vi "SubTest Monitor - GTCP331-200ER.vi"(8 "error in (no error)":errorcluster, 11 "RT - Analysis Data in in":T1={"Accel Sensistivity"=[0.0, 0.0, 0.0], "Cutoff Frequncies"=[{"LP Passband"=0.0, "HP Stopband"=0.0, "LP Stopband"=0.0, "HP Passband"=0.0}, {"LP Passband"=0.0, "HP Stopband"=0.0, "LP Stopband"=0.0, "HP Passband"=0.0}, {"LP Passband"=0.0, "HP Stopband"=0.0, "LP Stopband"=0.0, "HP Passband"=0.0}], "APU Setup File"={"Sensor Info"=[], "Calibration Info"=[], "CMM Table 106"=[], "CMM Table 106B "=[], "Accel Config"=[], "Report Sheet 1"=[], "Report Sheet 2"=[], "Report Sheet 3"=[]}, "RepairLevel"=""} {"Cutoff Frequncies"."HP Passband" min=1.0 step=1.0 format="%#.4f"; "Cutoff Frequncies"."LP Stopband" min=1.0 step=1.0 format="%#.4f"; "Cutoff Frequncies"."HP Stopband" min=1.0 step=1.0 format="%#.4f"; "Cutoff Frequncies"."LP Passband" min=1.0 step=1.0 format="%#.4f"}) -> (0 "error out":errorcluster, 3 "RT - Analysis Data out":T1 {"Cutoff Frequncies"."HP Passband" min=1.0 step=1.0 format="%#.4f"; "Cutoff Frequncies"."LP Stopband" min=1.0 step=1.0 format="%#.4f"; "Cutoff Frequncies"."HP Stopband" min=1.0 step=1.0 format="%#.4f"; "Cutoff Frequncies"."LP Passband" min=1.0 step=1.0 format="%#.4f"})   [LabVIEW 2018, in "RT - Analysis.lvlib"]
doc: "Monitors the data for the input SubTest for the named APU."
uses:
  RT - Analysis.lvlib
  Private Controls/RT-Analysis Data.ctl
  Modules/Testing UI 3/Private Controls/Cutoff Frequency.ctl
  Modules/Testing UI 3/Testing UI 3.lvlib
  Top Level/Shared Controls/APU Setup File.ctl
panel:
  # "Highpass Cutoff Frequency"
  # "Lowpass Cutoff Frequency"
  # "Highpass Cutoff Frequency"
  # "Lowpass Cutoff Frequency"
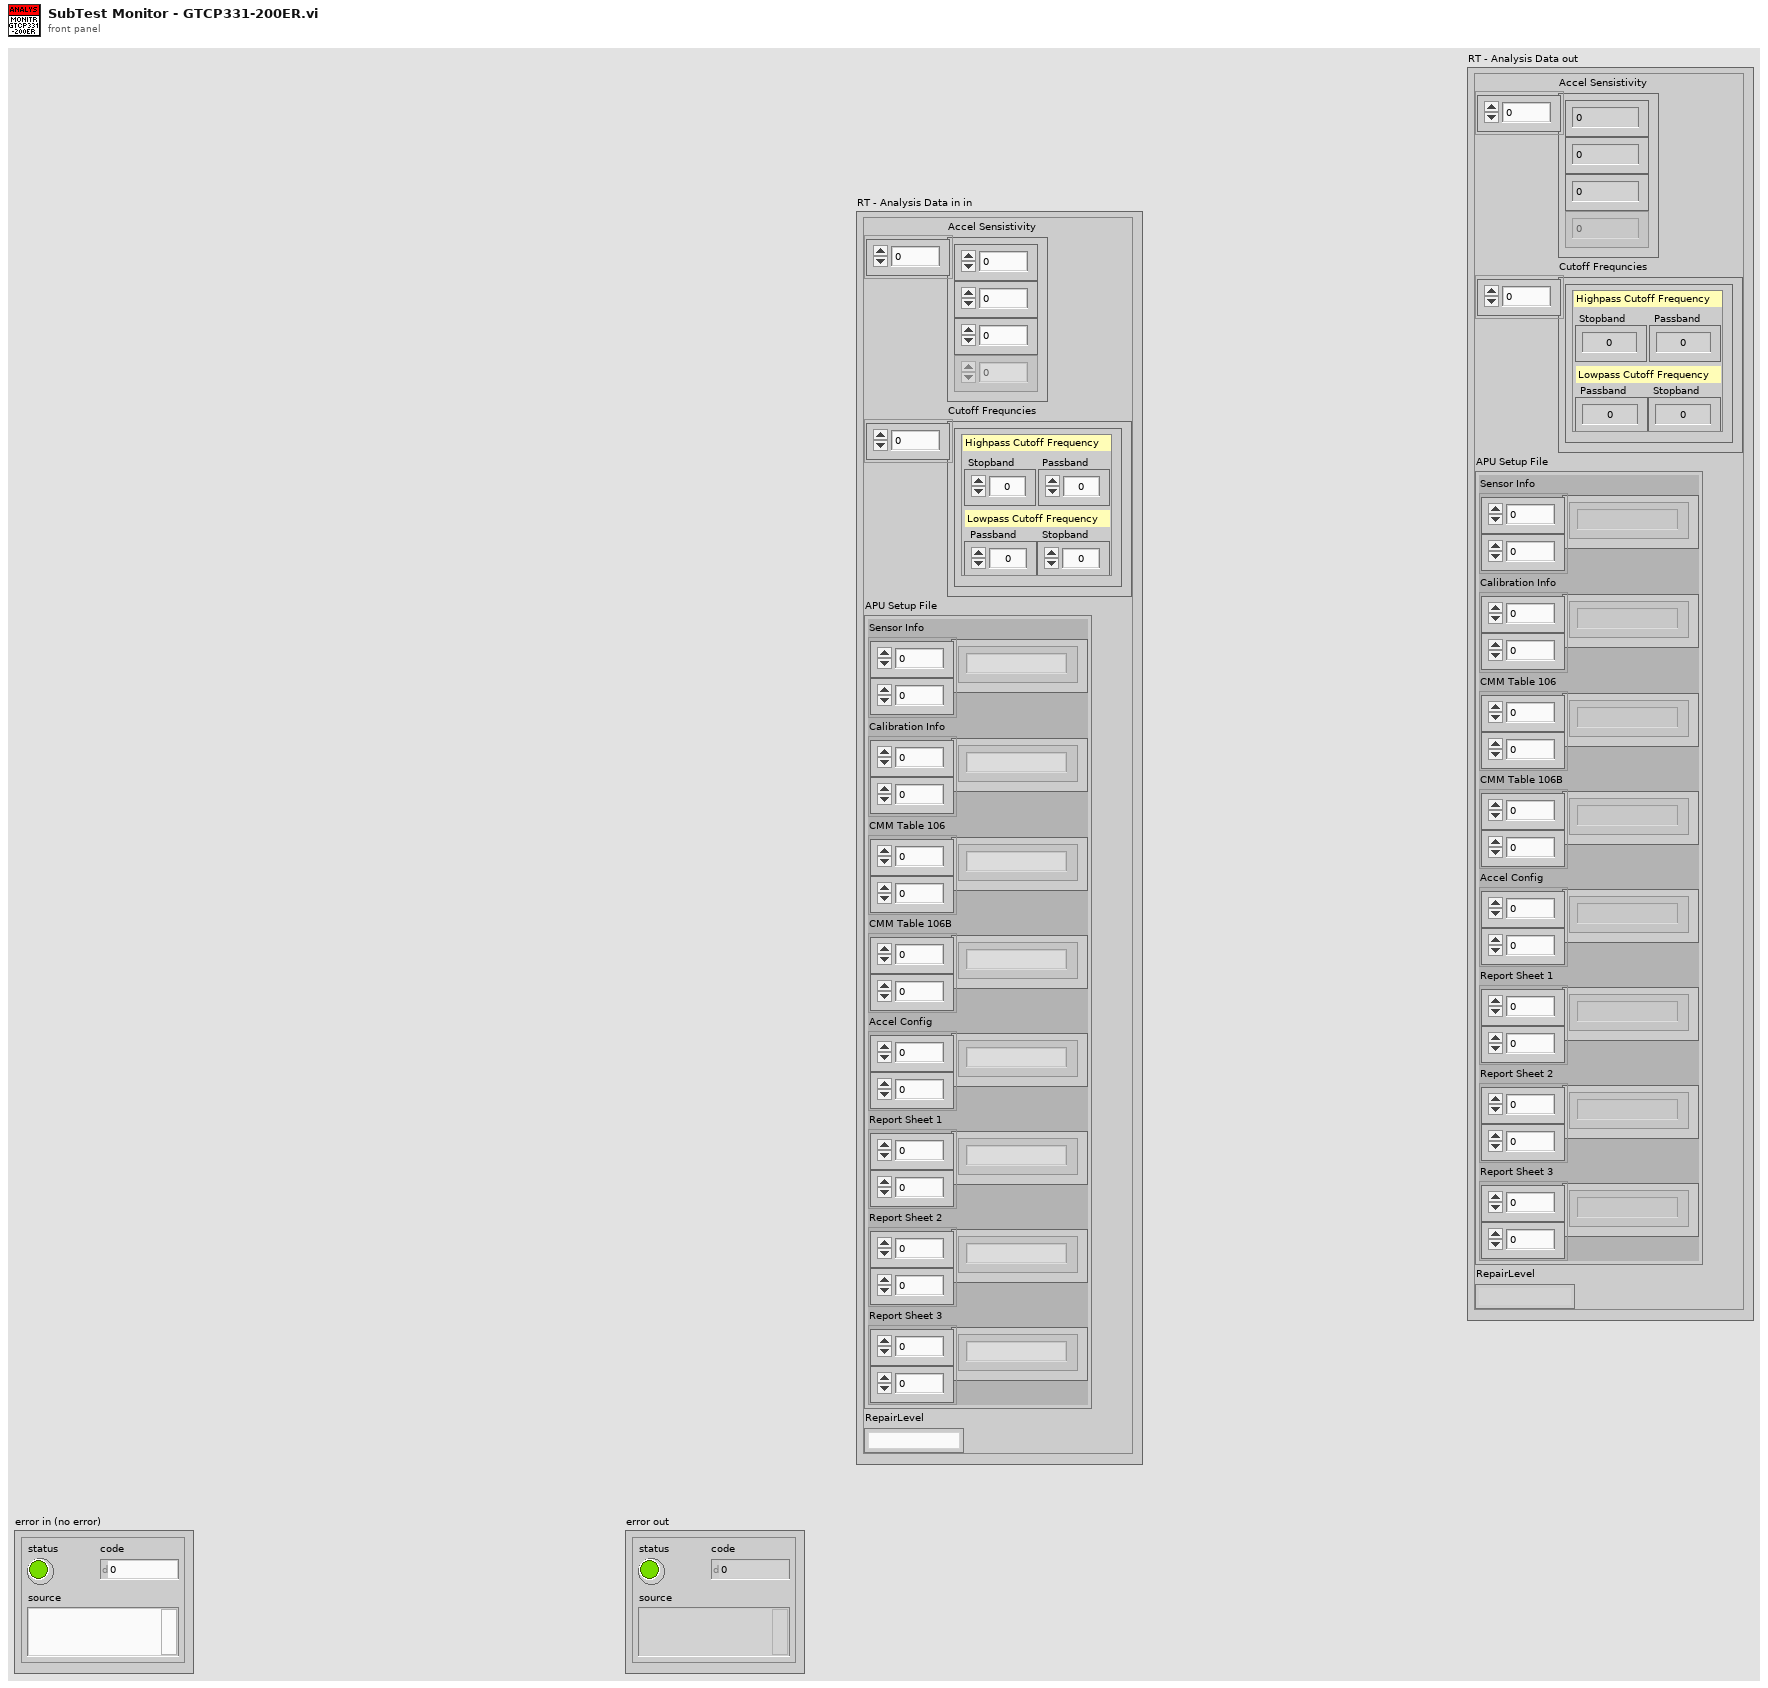
[diagram p1: front panel]
types:
  T1 = typedef "RT - Analysis.lvlib/RT-Analysis Data.ctl" = cluster{"Accel Sensistivity":dbl[], "Cutoff Frequncies":T2[], "APU Setup File":T3, "RepairLevel":string}
  T2 = typedef "Testing UI 3.lvlib/Cutoff Frequency.ctl" = cluster{"LP Passband":dbl, "HP Stopband":dbl, "LP Stopband":dbl, "HP Passband":dbl}
  T3 = typedef "APU Setup File.ctl" = cluster{"Sensor Info":string[][], "Calibration Info":string[][], "CMM Table 106":string[][], "CMM Table 106B ":string[][], "Accel Config":string[][], "Report Sheet 1":string[][], "Report Sheet 2":string[][], "Report Sheet 3":string[][]}
  T4 = typedef "Analyzed Data Sets.ctl" = T5[]
  T5 = typedef "All Data Cluster.ctl" = cluster{"Acq Data":T6, "Calculated Data":T7, "Indicator Data":cluster{"00-02-9234 Peak Vel (in/sec)":dbl[]}, "Calibrated Data":cluster{"00-00-9220 Calib":dbl[], "00-01-9220 Calib":dbl[], "02-03-9227 Calib":dbl[], "00-02-9234 Calib":dbl[], "02-05-9205 Calib":dbl[]}}
  T6 = typedef "Acq Data.ctl" = cluster{"00-00-9220":dbl[], "00-01-9220":dbl[], "01-00-9213":dbl[], "01-01-9213":dbl[], "01-02-9213":dbl[], "02-02-9219":dbl[], "02-03-9227":dbl[], "00-02-9234":dbl[], "00-03-9402":dbl[], "02-05-9205":dbl[], "02-04-9871":dbl[], "Timestamp":timestamp}
  T7 = typedef "Calculated Data.ctl" = cluster{"C.00":dbl, "C.01":dbl, "C.02":dbl, "C.03":dbl, "C.04":dbl, "C.05":dbl, "C.06":dbl, "C.07":dbl, "C.08":dbl, "C.09":dbl, "C.10":dbl, "C.11":dbl, "C.12":dbl, "C.13":dbl, "C.14":dbl, "C.15":dbl, "C.16":dbl, "C.17":dbl, "C.18":dbl, "C.19":dbl, "C.20":dbl, "C.21":dbl, "C.22":dbl, "C.23":dbl, "C.24":dbl, "C.25":dbl, "C.26":dbl, "C.27":dbl, "C.28":dbl, "C.29":dbl, "C.30":dbl, "C.31":dbl, "C.32":dbl, "C.33":dbl, "C.34":dbl, "C.35":dbl, "C.36":dbl, "C.37":dbl, "C.38":dbl, "C.39":dbl, "C.40":dbl, "C.41":dbl, "C.42":dbl, "C.43":dbl, "C.44":dbl, "C.45":dbl, "C.46":dbl, "C.47":dbl, "C.48":dbl, "C.49":dbl, "C.50":dbl, "C.51":dbl, "C.52":dbl, "C.53":dbl, "C.54":dbl, "C.56":dbl}
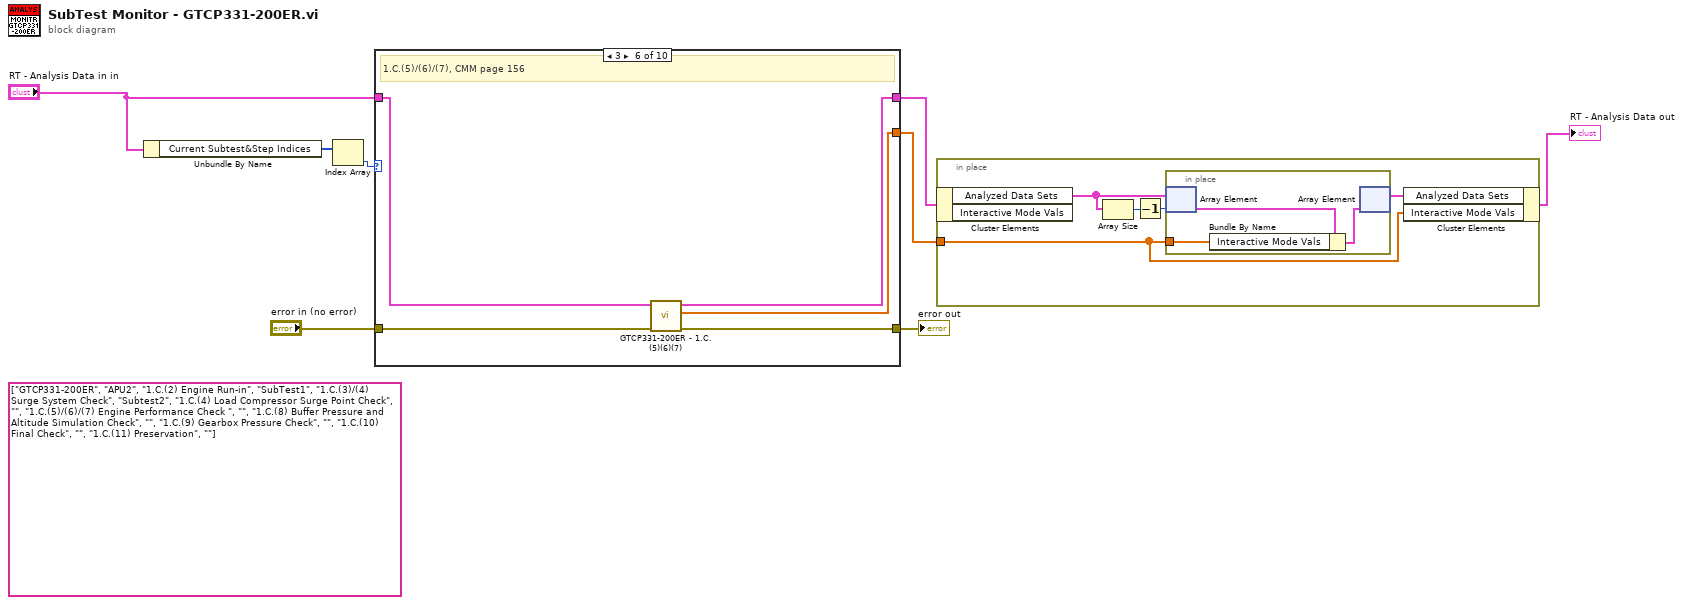
[diagram p0: block diagram]
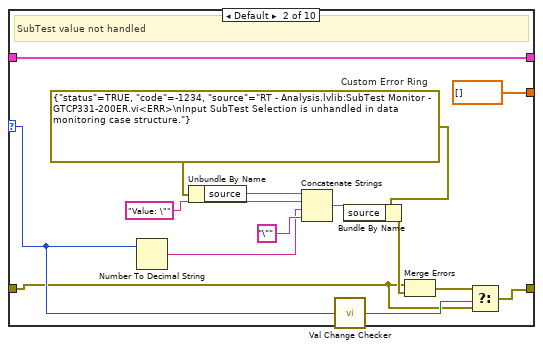
[diagram p3: hidden frame]
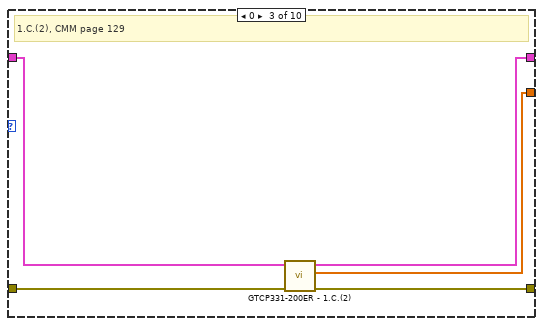
[diagram p4: hidden frame]
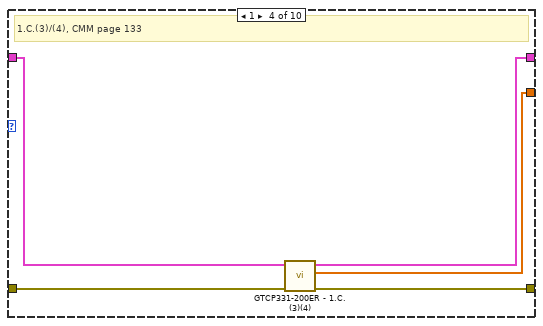
[diagram p5: hidden frame]
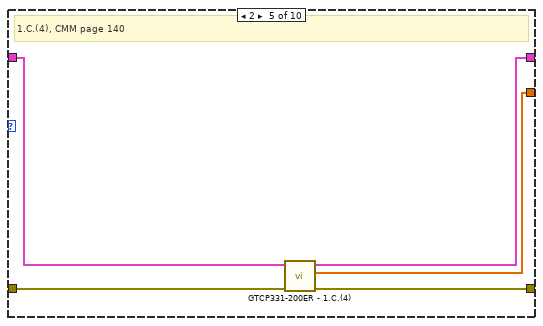
[diagram p6: hidden frame]
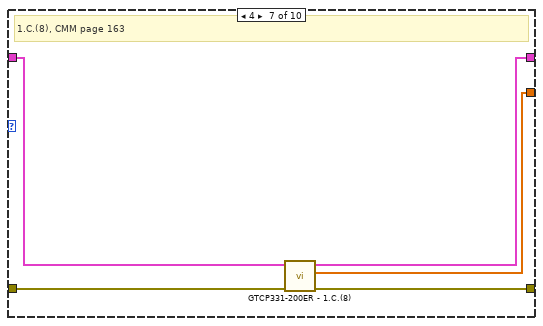
[diagram p7: hidden frame]
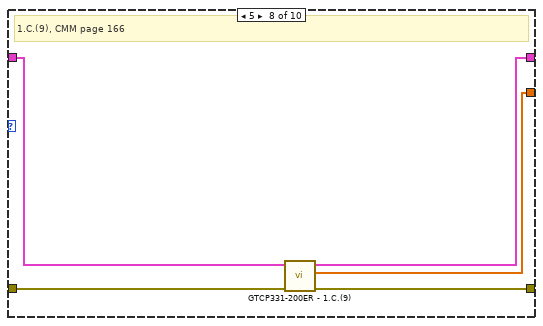
[diagram p8: hidden frame]
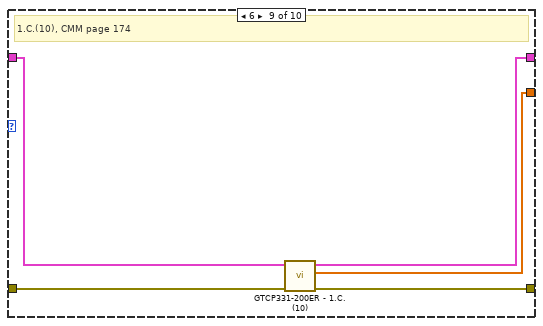
[diagram p9: hidden frame]
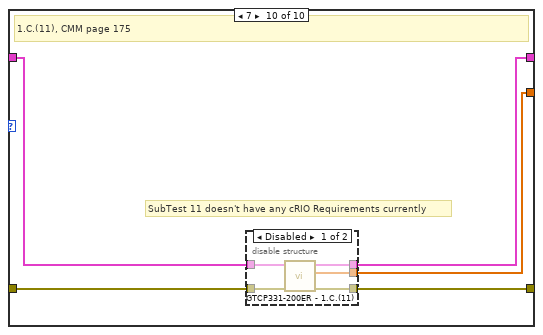
[diagram p10: hidden frame]
diagram:
  (unwired) string[][] [["GTCP331-200ER", "APU2"], ["1.C.(2) Engine Run-in", "SubTest1"], ["1.C.(3)/(4) Surge System Check", "Subtest2"], ["1.C.(4) Load Compressor Surge Point Check", ""], ["1.C.(5)/(6)/(7) Engine Performance Check ", ""], ["1.C.(8) Buffer Pressure and Altitude Simulation Check", ""], ["1.C.(9) Gearbox Pressure Check", ""], ["1.C.(10) Final Check", ""], ["1.C.(11) Preservation", ""]] ("APU Test Array")
  n1 = Unbundle By Name("RT - Analysis Data in in") -> ("Current Subtest&Step Indices"=w6:i32[])
  n2 = Index Array(array=w6) -> (element=w5:i32)  [unwired: 1 in]
  n3 = case shown="3" w5 {
    selector: w5 -> [_ w14 _ _ _ _ _ _ _ _]
    tunnel: "RT - Analysis Data in in" -> [w10 w24 w26 w30 w39 w44 w46 w51 w56 w61]
    tunnel: [w10 w24 w27 w31 w35 w43 w47 w52 w57 w62] -> w3
    tunnel: "error in (no error)" -> [w9 w11 w29 w34 w38 w41 w49 w54 w59 w64]
    tunnel: [w9 w15 w28 w33 w37 w40 w48 w53 w58 w63] -> w8
    tunnel: [_ dbl[] [] ("Interactive Mode Vals") w25 w32 w36 w42 w45 w50 w55 w60] -> w2
    frame -2, -1 {
      # "Do nothing when not in subtest"
    }
    frame Default {
      w17 = errorcluster {"status"=TRUE, "code"=-1234, "source"="RT - Analysis.lvlib:SubTest Monitor - GTCP331-200ER.vi<ERR>\nInput SubTest Selection is unhandled in data monitoring case structure."}  # Custom Error Ring
      # "SubTest value not handled"
      n4 = Number To Decimal String(number=w14) -> (decimal integer string=w16:string)  [unwired: 1 in]
      n5 = Unbundle By Name(w17) -> ("source"=w21:string)
      n6 = Concatenate Strings(w21, "Value: \"" ("string"), w16, "\"" ("string")) -> (w20:string)
      n7 = call "Val Change Checker.vi"("Current Value in"=w14) -> ("Value Change?"=w13:bool)
      n8 = Bundle By Name(cluster=w17, "source"=w20) -> (w22:errorcluster)
      n9 = Merge Errors(w11, w22) -> (w12:errorcluster)
      n10 = Select(t=w12, s=w13, f=w11) -> (s? t:f=w15:errorcluster)
    }
    frame 0 {
      # "1.C.(2), CMM page 129"
      n11 = call "GTCP331-200ER - 1.C.(2).vi"("error in (no error)"=w29, "RT - Analysis Data in in in"=w26) -> ("error out"=w28:errorcluster, "Interactive Mode Vals"=w25:dbl[], "RT - Analysis Data in out"=w27:T1)  [unwired: 7 in]
    }
    frame 1 {
      # "1.C.(3)/(4), CMM page 133"
      n12 = call "GTCP331-200ER - 1.C.(3)(4).vi"("error in (no error)"=w34, "RT - Analysis Data in in in"=w30) -> ("error out"=w33:errorcluster, "Interactive Mode Vals"=w32:dbl[], "RT - Analysis Data in out"=w31:T1)  [unwired: 7 in]
    }
    frame 2 {
      # "1.C.(4), CMM page 140"
      n13 = call "GTCP331-200ER - 1.C.(4).vi"("error in (no error)"=w38, "RT - Analysis Data in in in"=w39) -> ("error out"=w37:errorcluster, "Interactive Mode Vals"=w36:dbl[], "RT - Analysis Data in out"=w35:T1)  [unwired: 7 in]
    }
    frame 3 {
      # "1.C.(5)/(6)/(7), CMM page 156"
      n14 = call "GTCP331-200ER - 1.C.(5)(6)(7).vi"("error in (no error)"=w41, "RT - Analysis Data in in in"=w44) -> ("error out"=w40:errorcluster, "Interactive Mode Vals"=w42:dbl[], "RT - Analysis Data in out"=w43:T1)  [unwired: 7 in]
    }
    frame 4 {
      # "1.C.(8), CMM page 163"
      n15 = call "GTCP331-200ER - 1.C.(8).vi"("error in (no error)"=w49, "RT - Analysis Data in in in"=w46) -> ("error out"=w48:errorcluster, "Interactive Mode Vals"=w45:dbl[], "RT - Analysis Data in out"=w47:T1)  [unwired: 7 in]
    }
    frame 5 {
      # "1.C.(9), CMM page 166"
      n16 = call "GTCP331-200ER - 1.C.(9).vi"("error in (no error)"=w54, "RT - Analysis Data in in in"=w51) -> ("error out"=w53:errorcluster, "Interactive Mode Vals"=w50:dbl[], "RT - Analysis Data in out"=w52:T1)  [unwired: 7 in]
    }
    frame 6 {
      # "1.C.(10), CMM page 174"
      n17 = call "GTCP331-200ER - 1.C.(10).vi"("error in (no error)"=w59, "RT - Analysis Data in in in"=w56) -> ("error out"=w58:errorcluster, "Interactive Mode Vals"=w55:dbl[], "RT - Analysis Data in out"=w57:T1)  [unwired: 7 in]
    }
    frame 7 {
      # "SubTest 11 doesn't have any cRIO Requirements currently"
      # "1.C.(11), CMM page 175"
      n18 = disable-structure shown="Disabled" {
        disable-tunnel: w64 -> [w69 w70]
        disable-tunnel: [w68 w70] -> w63
        disable-tunnel: [w67 w71] -> w62
        disable-tunnel: w61 -> [w66 w71]
        disable-tunnel: [w65 _] -> w60
        frame Disabled {
          n19 = call "GTCP331-200ER - 1.C.(11).vi"("error in (no error)"=w69, "RT - Analysis Data in in in"=w66) -> ("error out"=w68:errorcluster, "Interactive Mode Vals"=w65:dbl[], "RT - Analysis Data in out"=w67:T1)  [unwired: 7 in]
        }
        frame Enabled {
        }
      }
    }
  }
  "error out" <- w8
  n20 = in-place {
    in-place-border: w2 -> [w72]
    n21 = in-place-cluster #1(w3) -> ("Analyzed Data Sets"=w75:T4)  [unwired: 1 out]
    n22 = Array Size(array=w75) -> (size(s)=w76:i32)
    n23 = Decrement(x=w76) -> (x-1=w74:i32)
    n24 = in-place {
      in-place-border: w72 -> [w77]
      n25 = in-place-array #2(w75, w74) -> (w79:T5)
      n26 = Bundle By Name(cluster=w79, "Interactive Mode Vals"=w77) -> (w78:T5)
      n27 = in-place-array #2(w78) -> (w73:T4)  [unwired: 1 out]
    }
    n28 = in-place-cluster #1("Analyzed Data Sets"=w73, "Interactive Mode Vals"=w72) -> (→"RT - Analysis Data out":T1)
  }
